vi "get_instances.vi"(6 "id (unnamed)":string, 8 "error in (no error)":errorcluster, 10 "Base Class (LabVIEW Object)":refnum<class>, 11 "Mapped Lookup in":refnum<class "Mapped Lookup.lvclass">) -> (0 "error out":errorcluster, 2 "instances":set{refnum<data-value>}(c389), 3 "Mapped Lookup out":refnum<class "Mapped Lookup.lvclass">)   [LabVIEW 2019, in "Lookup API.lvlib" / "Mapped Lookup.lvclass"]
doc: "<b>Description</b> Returns a set of instances of the specified <b>Base Class</b>."
uses:
  Mapped Lookup.lvclass
  Mapped Lookup.lvclass/Mapped Lookup.ctl
  4ca94fd0-0d33-4777-823f-87de04f59e78.vi
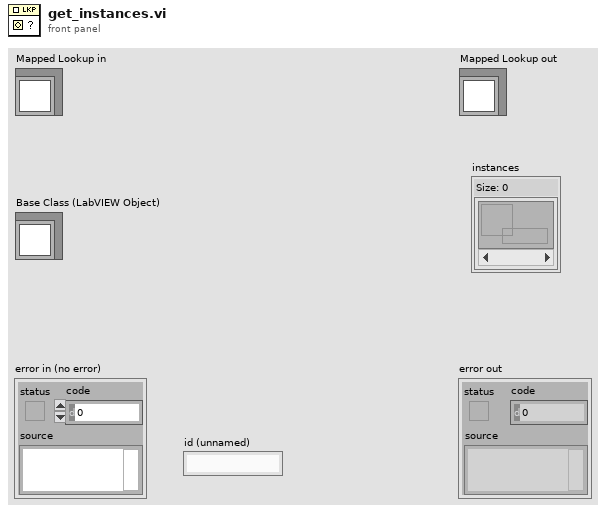
[diagram p1: front panel]
types:
  T1 = map{string, cluster{"instances":refnum<data-value>, "events":refnum<data-value>}}
  T2 = cluster{"instances":refnum<data-value>, "events":refnum<data-value>}
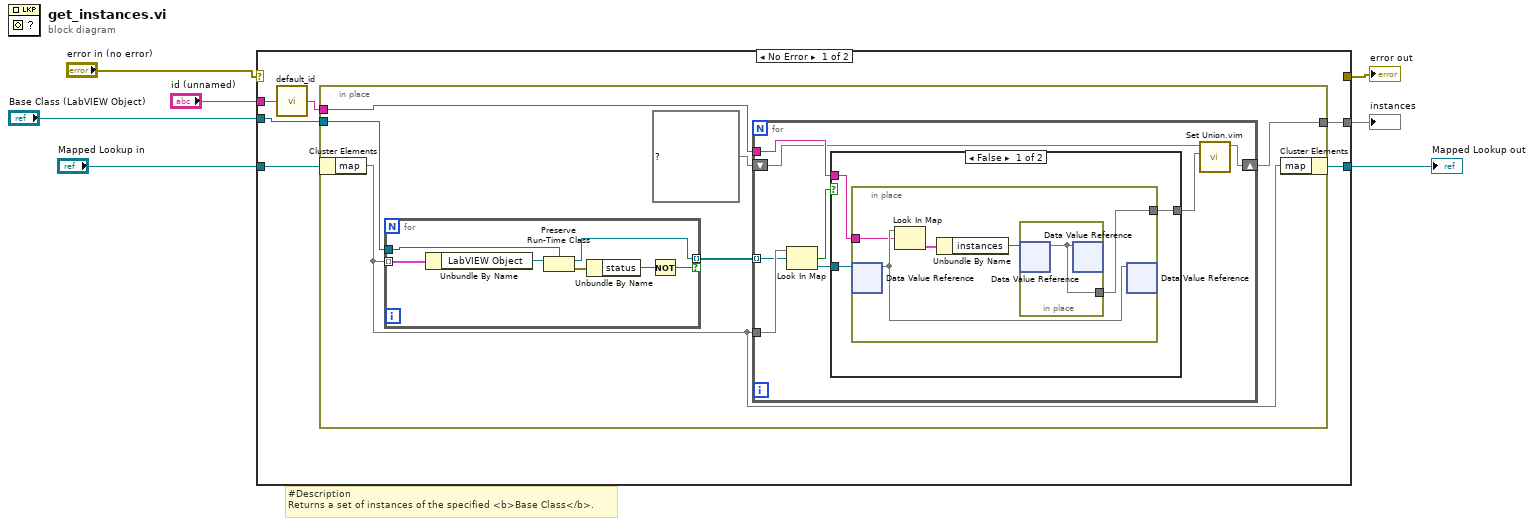
[diagram p0: block diagram]
diagram:
  # "#Description\nReturns a set of instances of the specified <b>Base Class</b>."
  n1 = case shown="No Error" "error in (no error)" {
    selector: "error in (no error)" -> [_ w45]
    tunnel: [_ w45] -> w6
    tunnel: [w10 w44] -> w5
    tunnel: "Mapped Lookup in" -> [w12 w44]
    tunnel: "id (unnamed)" -> [w13 _]
    tunnel: "Base Class (LabVIEW Object)" -> [w11 _]
    tunnel: [w8 _] -> w1
    frame No Error {
      n2 = call "default_id.vi"("id (unnamed)"=w13) -> ("String"=w9:string)
      n3 = in-place {
        in-place-border: w11 -> [w16]
        in-place-border: w9 -> [w19]
        in-place-border: [w18] -> w8
        n4 = in-place-cluster #1(w12) -> ("map"=w17:map{refnum<class>, refnum<data-value>})
        n5 = for {
          tunnel: w17 -> [w43] mode=indexing
          tunnel: w16 -> [w42]
          tunnel: [w40] -> w15 mode=indexing if=w37
          n6 = Unbundle By Name(w43) -> ("LabVIEW Object"=w41:refnum<class>)
          n7 = Preserve Run-Time Class(object in=w41, 2:w42) -> (object out=w40:refnum<class>, error out=w39:errorcluster)  [unwired: 1 in]
          n8 = Unbundle By Name(w39) -> ("status"=w38:bool)
          n9 = Not(x=w38) -> (.not. x?=w37:bool)
        }
        n10 = for {
          tunnel: w19 -> [w25]
          tunnel: w17 -> [w24]
          tunnel: w15 -> [w23] mode=indexing
          shift-right: [w20] -> w18
          shift-left: set{refnum<data-value>} {} ("set") -> [w22]
          n11 = Look In Map(map=w24, key=w23) -> (key not found?=w27:bool, value=w26:refnum<data-value>)  [unwired: 1 in]
          n12 = case shown="False" w27 {
            tunnel: w26 -> [w30 _]
            tunnel: w25 -> [w29 _]
            tunnel: [w28 _] -> w21
            frame False {
              n13 = in-place {
                in-place-border: w29 -> [w34]
                in-place-border: [w31] -> w28
                n14 = in-place-dvr #2(w30) -> (w35:T1)  [unwired: 1 out]
                n15 = Look In Map(map=w35, key=w34) -> (value=w33:T2)  [unwired: 1 in, 1 out]
                n16 = Unbundle By Name(w33) -> ("instances"=w32:refnum<data-value>)
                n17 = in-place {
                  in-place-border: [w36] -> w31
                  n18 = in-place-dvr #3(w32) -> (w36:set{refnum<data-value>})  [unwired: 1 out]
                  n19 = in-place-dvr #3(w36) -> ()  [unwired: 2 out]
                }
                n20 = in-place-dvr #2(w35) -> ()  [unwired: 2 out]
              }
            }
            frame True {
            }
          }
          n21 = call "Set Union.vim"("set 2"=w21, "set 1"=w22) -> ("union"=w20:set{refnum<data-value>})  [unwired: 9 in]
        }
        n22 = in-place-cluster #1("map"=w17) -> (w10:refnum<class "Mapped Lookup.lvclass">)
      }
    }
    frame Error {
    }
  }
  "error out" <- w6
  "Mapped Lookup out" <- w5
  "instances" <- w1
